vi "SMC GenEvent= Message.vi"(0 "Event Number":dbl) -> ()   [LabVIEW 2010]
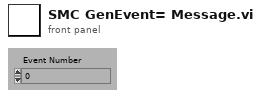
[diagram p1: front panel]
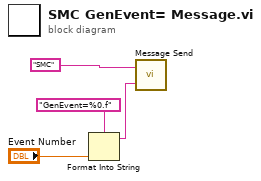
[diagram p0: block diagram]
diagram:
  n1 = Format Into String(format string="GenEvent=%0.f", "Event Number") -> (resulting string=w3:string)  [unwired: 2 in, 1 out]
  n2 = call "Message Send.vi"("Message"=w3, "Destination"="SMC" ("Destination(s)")) -> ()
